vi "SYSID_FPGA.vi"() -> ()   [LabVIEW 2014, in "SYSID.lvlib"]
doc: "This VI was generated automatically using the FPGA Wizard. You can modify the VI normally."
uses:
  SYSID.lvlib
  <vilib>/Platform/TimedLoop/XDataNode/timing_clust.ctl
  <vilib>/Platform/TimedLoop/XDataNode/nitl_modes.ctl
  <vilib>/Platform/TimedLoop/XDataNode/wakeup.ctl
  <vilib>/rvi/FXPMathLib/FxpConvert/subVIs/nifxpmath_Convert_SimConfig.ctl
  <vilib>/fxp/LVFixedPointQuantizationPolicyTypeDef.ctl
  <vilib>/fxp/LVFixedPointOverflowPolicyTypeDef.ctl
  <vilib>/rvi/Emulation/niFpgaGetClockAttributes.vi
  <vilib>/rvi/Emulation/niFpgaSctlEmulationGetInTimedLoop.vi
  <vilib>/rvi/Emulation/niFpgaEmulationReportErrorSimple.vi
  <vilib>/rvi/Emulation/niFpgaCriticalErrorInLSC.vi
  <vilib>/rvi/Emulation/niFpgaProcessEmulError.vi
  <vilib>/rvi/eio/common/nirviEmuTemplateMethod_errors.vi
  <vilib>/rvi/FXPMathLib/FxpConvert/simVIs/DllFxpConvertTemp_sub.vi
  <vilib>/Platform/TimedLoop/XDataNode/XDataNode.xnode
  <vilib>/eio/EIONode/EIONode.xnode
  <vilib>/rvi/FXPMathLib/FxpSub/XNode/nifxpmath_Sub.xnode
  <vilib>/rvi/FXPMathLib/FxpMul/XNode/nifxpmath_Multiplier.xnode
  <vilib>/rvi/FXPMathLib/FxpAdd/XNode/nifxpmath_Add.xnode
  <vilib>/rvi/FXPMathLib/FxpConvert/XNode/nifxpmath_Convert.xnode
  <vilib>/Platform/TimedLoop/XDataNode/XDNodeRunTimeDep.lvlib
  <vilib>/rvi/FXPMathLib/sim/FxpSim.dll
panel:
  out "Amp Cpmmand":fxp<+/-,20,5>
  in  "Reference":i32
  out "Right Limit":bool
  out "Left Limit":bool
  in  "Brake":bool=TRUE
  in  "Amp Reset":bool=TRUE
  in  "Amp Enable":bool
  in  "DGain":fxp<+/-,32,7>
  in  "PGain":fxp<+/-,32,7>
  out "Error-dot":fxp<+/-,55,34>
  out "Error":fxp<+/-,33,33>
  out "Control Late? (Latched)":bool
  out "Actual Control Rate (Ticks)":u32
  in  "Control Reset":bool
  in  "Control Rate (ticks)":u32=1000 caption="Control Rate (Ticks)"
  out "quad saved (Port0/DIO0,Port0/DIO1)":cluster{"Position":i32, "Index Count":u16}
  out "quad pos (Port0/DIO0,Port0/DIO1)":i32
  out "_quad pos (Port0/DIO0,Port0/DIO1)":i32
  in  "quad reset (Port0/DIO0,Port0/DIO1)":bool
  out "_quad saved (Port0/DIO0,Port0/DIO1)":cluster{"Position":i32, "Index Count":u16}
  in  "AO (ModB/AO2)":fxp<+/-,20,5>
  in  "AO (ModB/AO1)":fxp<+/-,20,5>
  out "AI (ModA/AI0)":fxp<+/-,26,5> format="%.6g"
  in  "Local Stop 0":bool
  out "Actual Loop Rate (Ticks)":u32
  out "Late? Latched":bool
  in  "Loop Rate (Ticks)":u32=571
  in  "Reset":bool
  in  "Start 0":bool
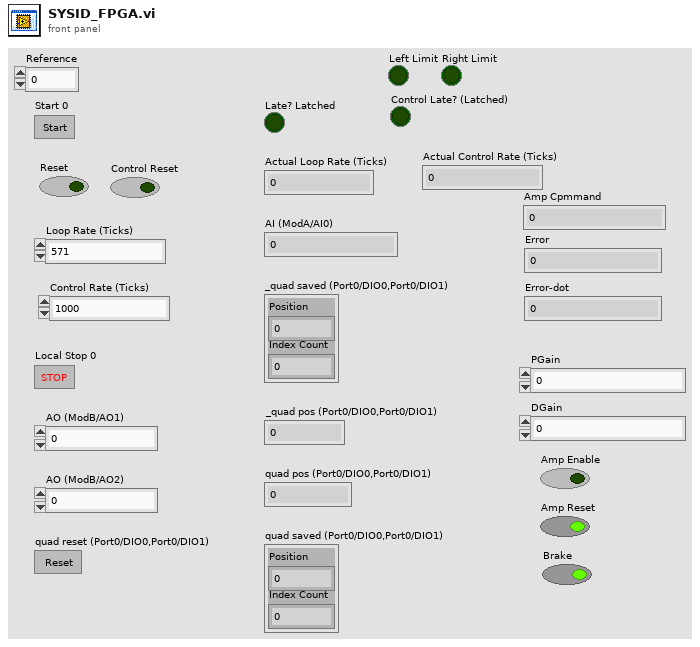
[diagram p1: front panel]
types:
  T1 = typedef "XDNodeRunTimeDep.lvlib/timing_clust.ctl" = cluster{"Expected End [f-1]":u64, "Actual End [f-1]":u64, "Finished Late? [f-1]":bool, "Expected End [i-1]":u64, "Actual End [i-1]":u64, "Finished Late? [i-1]":bool, "Expected Start [i]":u64, "Actual Start [i]":u64, "Expected Start [f]":u64, "Actual Start [f]":u64, "Source Name":string, "Structure Name":string, "Period":i64, "Deadline":i64, "Offset":i64, "Start":i64, "Priority":i32, "Timeout":i32, "Mode":T2, "Wakeup Reason":T3, "Error":errorcluster, "Source Type":string, "Secondary Source Type":string, "Global End Time":u64, "Global Start Time":u64, "Frame Duration":u64, "Iteration Duration":u64, "Assigned CPU":i32, "I/O Scan Engine Mode":u32}
  T2 = typedef "XDNodeRunTimeDep.lvlib/nitl_modes.ctl" = enum32{"No Change", "Process missed periods, maintain original phase", "Discard missed periods, maintain original phase", "Process missed periods, ignore original phase", "Discard missed periods, ignore original phase"}
  T3 = typedef "XDNodeRunTimeDep.lvlib/wakeup.ctl" = enum32{"Normal", "Aborted", "Asynchronous wakeup", "Timing source error", "Timed loop error", "Timeout"}
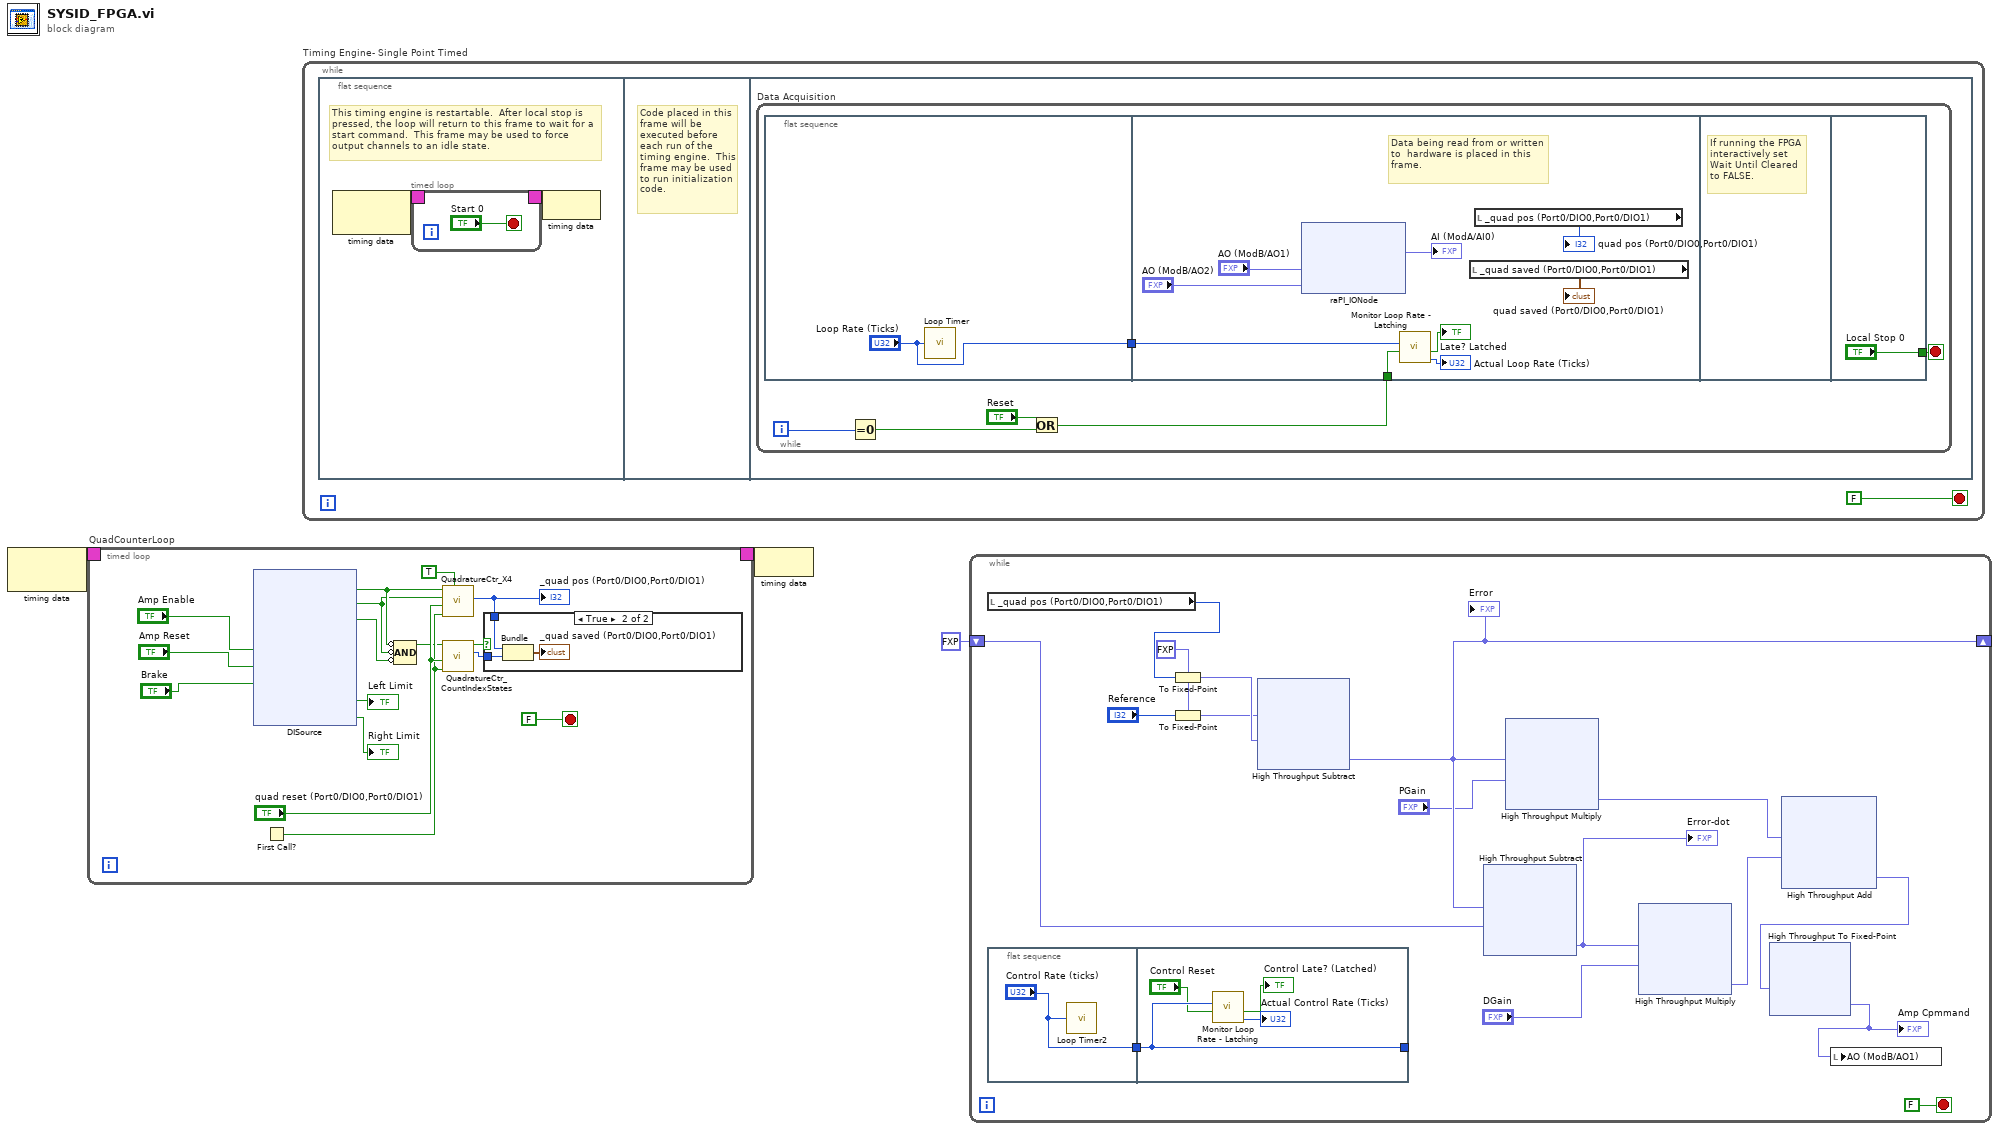
[diagram p0: block diagram]
diagram:
  n1 = node-c288 ("Input Node")() -> (w3:T1)  [unwired: 1 in]
  n2 = timed-loop "QuadCounterLoop" {
    timing: w3 -> [_]
    timing-out: [_] -> w2
    stop <- FALSE stop-if-true
    n3 = xnode ("DISource")("Port0/DIO6"="Amp Enable", "Port0/DIO7"="Amp Reset", "Port0/DIO5"="Brake") -> ("Port0/DIO0"=w12:bool, "Port0/DIO1"=w11:bool, "Port0/DIO2"=w10:bool, "Port0/DIO8"=→"Left Limit":bool, "Port0/DIO4"=→"Right Limit":bool)  [unwired: 8 in, 8 out]
    n4 = First Call?() -> (First Call?: T/F=w15:bool)
    n5 = Compound Arithmetic op=AND(invert w12, invert w11, invert w10) -> (w9:bool)
    n6 = call "QuadratureCtr_X4.vi"("Direction?"=TRUE, "First Run?"=w15, "Reset"="quad reset (Port0/DIO0,Port0/DIO1)", "Source B"=w11, "Source A"=w12) -> ("Position"=w17:i32)  [unwired: 6 in]
    "_quad pos (Port0/DIO0,Port0/DIO1)" <- w17
    n7 = call "QuadratureCtr_CountIndexStates.vi"("First Run?"=w15, "Reset"="quad reset (Port0/DIO0,Port0/DIO1)", "Valid Index State?"=w9) -> ("Index State Count"=w14:u16, "Save State?"=w13:bool)  [unwired: 7 in]
    n8 = case shown="True" w13 {
      tunnel: w17 -> [_ w22]
      tunnel: w14 -> [_ w20]
      frame False {
      }
      frame True {
        n9 = Bundle("Position"=w22, "Index State Count"=w20) -> (→"_quad saved (Port0/DIO0,Port0/DIO1)":cluster{"Position":i32, "Index State Count":u16})  [unwired: 1 in]
      }
    }
  }
  n10 = while "Timing Engine- Single Point Timed" {
    stop <- FALSE stop-if-true
    n11 = flat-sequence "MainSeq" {
      frame #0 {
        # "This timing engine is restartable.  After local stop is pressed, the loop will return to this frame to wait for a start command.  This frame may be used to force output channels to an idle state."
        n12 = node-c288 ("Input Node")() -> (w27:T1)  [unwired: 1 in]
        n13 = timed-loop "initWait" {
          timing: w27 -> [_]
          timing-out: [_] -> w26
          stop <- "Start 0" stop-if-true
        }
        n14 = node-c288 ("Output Node")(w26) -> ()
      }
      frame #1 {
        # "Code placed in this frame will be executed before each run of the timing engine.  This frame may be used to run initialization code."
      }
      frame #2 {
        n15 = while "Data Acquisition" {
          i -> [w36]
          stop <- w38 stop-if-true
          n16 = flat-sequence "Data Acquisition Sequence" {
            tunnel: ["Loop Rate (Ticks)"] -> w37
            tunnel: w37 -> [w46]
            tunnel: w33 -> [w45]
            tunnel: ["Local Stop 0"] -> w38
            frame #0 {
              n17 = call "Loop Timer"("Count(Ticks)"="Loop Rate (Ticks)") -> ()  [unwired: 1 out]
            }
            frame #1 {
              # "Data being read from or written to  hardware is placed in this frame."
              n18 = xnode ("raPI_IONode")("ModB/AO0"="AO (ModB/AO1)", "ModB/AO2"="AO (ModB/AO2)") -> ("ModA/AI0"=→"AI (ModA/AI0)":fxp<+/-,26,5>)  [unwired: 3 in, 3 out]
              n19 = call "Monitor Loop Rate - Latching.vi"("Reset"=w45, "Count(Ticks)"=w46) -> ("Actual Loop Rate (Ticks)"=→"Actual Loop Rate (Ticks)":u32, "Late? (Latched)"=→"Late? Latched":bool)  [unwired: 7 in, 1 out]
              n20 = local read "_quad saved (Port0/DIO0,Port0/DIO1)"() -> (→"quad saved (Port0/DIO0,Port0/DIO1)":cluster{"Position":i32, "Index Count":u16})
              n21 = local read "_quad pos (Port0/DIO0,Port0/DIO1)"() -> (→"quad pos (Port0/DIO0,Port0/DIO1)":i32)
            }
            frame #2 {
              # "If running the FPGA interactively set Wait Until Cleared to FALSE."
            }
            frame #3 {
            }
          }
          n22 = Equal To 0?(x=w36) -> (x = 0?=w35:bool)
          n23 = Or(x="Reset", y=w35) -> (x .or. y?=w33:bool)
        }
      }
    }
  }
  n24 = node-c288 ("Output Node")(w2) -> ()
  n25 = while {
    shift-right: [w64] -> _
    shift-left: fxp<+/-,54,33> 0.0 ("x-y") -> [w63]
    stop <- FALSE stop-if-true
    w51 = fxp<+/-,32,32> 0.0 ("y")
    n26 = local read "_quad pos (Port0/DIO0,Port0/DIO1)"() -> (w65:i32)
    n27 = flat-sequence {
      tunnel: ["Control Rate (ticks)"] -> w60
      tunnel: [w70] -> _
      tunnel: w60 -> [w70]
      frame #0 {
        n28 = call "Loop Timer2"("Count(Ticks)"="Control Rate (ticks)") -> ()  [unwired: 1 out]
      }
      frame #1 {
        n29 = call "Monitor Loop Rate - Latching.vi"("Reset"="Control Reset", "Count(Ticks)"=w70) -> ("Actual Loop Rate (Ticks)"=→"Actual Control Rate (Ticks)":u32, "Late? (Latched)"=→"Control Late? (Latched)":bool)  [unwired: 7 in, 1 out]
      }
    }
    n30 = To Fixed-Point(fixed-point type=w51, number=w65) -> (fixed-point=w53:fxp<+/-,32,32>)
    n31 = To Fixed-Point(fixed-point type=w51, number="Reference") -> (fixed-point=w50:fxp<+/-,32,32>)
    n32 = xnode "High Throughput Subtract"("x"=w50, "y"=w53) -> ("x-y"=w64:fxp<+/-,33,33>)
    "Error" <- w64
    n33 = xnode "High Throughput Subtract"("x"=w64, "y"=w63) -> ("x-y"=w62:fxp<+/-,55,34>)
    "Error-dot" <- w62
    n34 = xnode "High Throughput Multiply"("x"=w64, "y"="PGain") -> ("x*y"=w58:fxp<+/-,64,40>)
    n35 = xnode "High Throughput Multiply"("x"=w62, "y"="DGain") -> ("x*y"=w57:fxp<+/-,64,41>)
    n36 = xnode "High Throughput Add"("x"=w58, "y"=w57) -> ("x+y"=w56:fxp<+/-,64,42>)
    n37 = xnode "High Throughput To Fixed-Point"("x"=w56) -> ("y"=w61:fxp<+/-,20,5>)
    "Amp Cpmmand" <- w61
    n38 = local write "AO (ModB/AO1)"(w61) -> ()
  }
